vi "Load Technique.vi"(8 "error in (no error)":errorcluster, 9 "Technique Parameters in":variant, 10 "Technique in":T1, 11 "Potentiostat Galvanostat in":refnum<class "Potentiostat Galvanostat.lvclass">) -> (0 "error out":errorcluster, 3 "Potentiostat Galvanostat out":refnum<class "Potentiostat Galvanostat.lvclass">)   [LabVIEW 2018, in "Potentiostat Galvanostat.lvclass"]
uses:
  Potentiostat Galvanostat.lvclass
  Controls/Technique List.ctl
  Potentiostat Galvanostat.lvclass/Potentiostat Galvanostat.ctl
  Error Code Converter.vi
  BL_GetErrorMsg.vi
  <vilib>/Utility/error.llb/Error Cluster From Error Code.vi
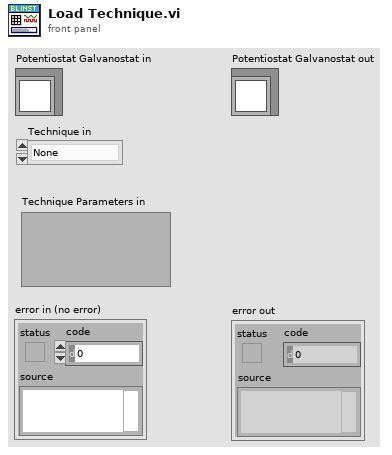
[diagram p1: front panel]
types:
  T1 = typedef "Potentiostat Galvanostat.lvclass/Technique List.ctl" = enum16{"None", "ocv", "cv", "biovscan", "ca", "cp", "iscan", "vscan", "lasv", "load", "pow", "peis", "geis", "seisp", "seisg", "dpv", "swv", "npv", "mpv", "dnpv", "dpa", "evt", "lp", "gc", "cpp", "pdp", "psp", "zra", "ircmp", "pzir", "gzir", "loop", "TO", "TI", "TOS", "vscanlimit", "iscanlimit", "mp", "casp", "casg", "calimit", "cplimit"}
  T2 = typedef "Potentiostat Galvanostat.lvclass/Technique Parameter.ctl" = cluster{"Parameter Label":string, "Parameter Type":T3, "Parameter Value":i32, "Parameter Index":i32}
  T3 = typedef "Potentiostat Galvanostat.lvclass/Parameter Type.ctl" = i32
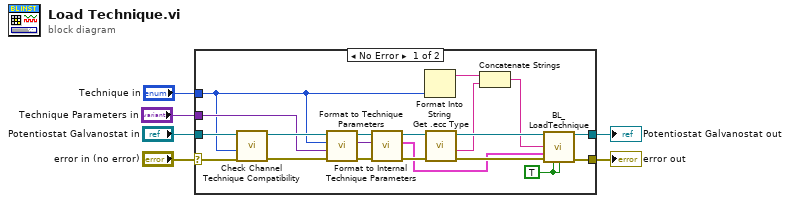
[diagram p0: block diagram]
diagram:
  n1 = case shown="No Error" "error in (no error)" {
    selector: "error in (no error)" -> [w22 w28]
    tunnel: [w20 w27] -> w4
    tunnel: "Potentiostat Galvanostat in" -> [w21 w27]
    tunnel: "Technique in" -> [w10 _]
    tunnel: "Technique Parameters in" -> [w11 _]
    tunnel: [w19 w28] -> w1
    frame No Error {
      w24 = TRUE ("FirstTechnique")
      n2 = call "Check Channel Technique Compatibility.vi"("error in (no error)"=w22, "Technique in"=w10, "Potentiostat Galvanostat in"=w21) -> ("error out"=w12:errorcluster, "Potentiostat Galvanostat out"=w13:refnum<class "Potentiostat Galvanostat.lvclass">)  [unwired: 6 in, 1 out]
      n3 = call "Format to Internal Technique Parameters.vi"("error in (no error)"=w12, "Technique Parameters (Typedefs)"=w11, "Technique"=w10, "Potentiostat Galvanostat in"=w13) -> ("error out"=w16:errorcluster, "Internal Technique Parameters"=w15:variant, "Potentiostat Galvanostat out"=w14:refnum<class "Potentiostat Galvanostat.lvclass">)  [unwired: 5 in]
      n4 = call "Format to Technique Parameters.vi"("error in (no error)"=w16, "Internal Technique Parameter"=w15, "Potentiostat Galvanostat in"=w14) -> ("error out"=w9:errorcluster, "Technique Parameters"=w7:T2[], "Potentiostat Galvanostat out"=w8:refnum<class "Potentiostat Galvanostat.lvclass">)  [unwired: 6 in]
      n5 = Format Into String(w10) -> (resulting string=w17:string)  [unwired: 3 in, 1 out]
      n6 = call "Get .ecc Type.vi"("error in (no error)"=w9, "Potentiostat Galvanostat in"=w8) -> ("error out"=w18:errorcluster, "Ecc Type"=w25:string, "Potentiostat Galvanostat out"=w26:refnum<class "Potentiostat Galvanostat.lvclass">)  [unwired: 6 in, 1 out]
      n7 = Concatenate Strings(w17, w25) -> (w23:string)
      n8 = call-dynamic "BL_LoadTechnique.vi"("Potentiostat Galvanostat in"=w26, "Technique File Name (.ecc)"=w23, "Technique Parameters"=w7, "error in (no error)"=w18, "FirstTechnique"=w24, "LastTechnique"=w24) -> ("Potentiostat Galvanostat out"=w20:refnum<class "Potentiostat Galvanostat.lvclass">, "error out"=w19:errorcluster)  [unwired: 7 in, 1 out]
    }
    frame Error {
    }
  }
  "error out" <- w1
  "Potentiostat Galvanostat out" <- w4
